vi "ClientForSingleDeviceDServer_05.vi"() -> ()   [LabVIEW 2014, in "examples.lvlib"]
uses:
  vis/tango_vi.llb/_DServerDevicePropertyToDouble.vi
  vis/tango_vi.llb/_DServerDevicePropertyToFloat.vi
  vis/tango_vi.llb/_DServerDevicePropertyToULong.vi
  vis/tango_vi.llb/_DServerDevicePropertyToLong.vi
  vis/tango_vi.llb/_DServerDevicePropertyToUShort.vi
  vis/tango_vi.llb/_DServerDevicePropertyToShort.vi
  vis/tango_vi.llb/_DServerDevicePropertyToBoolean.vi
  vis/tango_vi.llb/_DServerDevicePropertyToDoubleArray.vi
  vis/tango_vi.llb/_DServerDevicePropertyToFloatArray.vi
  vis/tango_vi.llb/_DServerDevicePropertyToShortArray.vi
  vis/tango_vi.llb/_DServerDevicePropertyToLongArray.vi
  vis/tango_vi.llb/_DServerDevicePropertyToString.vi
  vis/tango_vi.llb/_DServerDevicePropertyToStringArray.vi
  examples.lvlib
  vis/tango_vi.llb/tango.lvlib
panel:
  out "PropertyDevStringArray":string[](array[string])
  out "PropertyDevString":string
  out "PropertyDevLongArray":i32[](array[numeric])
  out "PropertyDevShortArray":i16[](array[numeric])
  out "PropertyDevFloatArray":dbl[](array[numeric])
  out "PropertyDevDoubleArray":dbl[](array[numeric])
  out "PropertyDevBoolean":bool=TRUE
  out "PropertyDevShort":i16
  out "PropertyDevUShort":u16
  out "PropertyDevLong":i32
  out "PropertyDevULong":u32
  out "PropertyDevFloat":sgl
  out "PropertyDevDouble":dbl
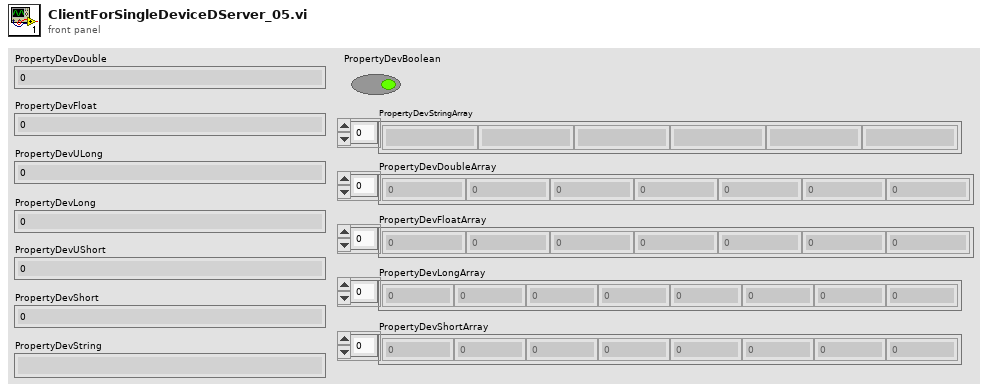
[diagram p1: front panel]
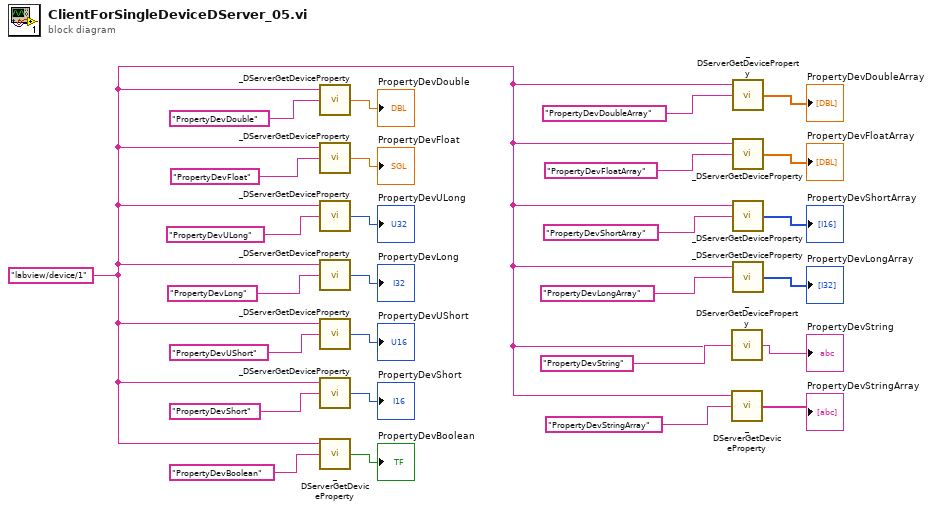
[diagram p0: block diagram]
diagram:
  w2 = "labview/device/1" ("device name")
  n1 = call-poly "_DServerGetDeviceProperty.vi"("property name"="PropertyDevDouble", "device name"=w2) -> ("property value"=→"PropertyDevDouble":dbl)  [unwired: 2 in, 1 out]
  n2 = call-poly "_DServerGetDeviceProperty.vi"("property name"="PropertyDevFloat", "device name"=w2) -> ("property value"=→"PropertyDevFloat":sgl)  [unwired: 2 in, 1 out]
  n3 = call-poly "_DServerGetDeviceProperty.vi"("property name"="PropertyDevULong", "device name"=w2) -> ("property value"=→"PropertyDevULong":u32)  [unwired: 2 in, 1 out]
  n4 = call-poly "_DServerGetDeviceProperty.vi"("property name"="PropertyDevLong", "device name"=w2) -> ("property value"=→"PropertyDevLong":i32)  [unwired: 2 in, 1 out]
  n5 = call-poly "_DServerGetDeviceProperty.vi"("property name"="PropertyDevUShort", "device name"=w2) -> ("property value"=→"PropertyDevUShort":u16)  [unwired: 2 in, 1 out]
  n6 = call-poly "_DServerGetDeviceProperty.vi"("property name"="PropertyDevShort", "device name"=w2) -> ("property value"=→"PropertyDevShort":i16)  [unwired: 2 in, 1 out]
  n7 = call-poly "_DServerGetDeviceProperty.vi"("property name"="PropertyDevBoolean", "device name"=w2) -> ("property value"=→"PropertyDevBoolean":bool)  [unwired: 2 in, 1 out]
  n8 = call-poly "_DServerGetDeviceProperty.vi"("property name"="PropertyDevString", "device name"=w2) -> ("propery value"=→"PropertyDevString":string)  [unwired: 2 in, 1 out]
  n9 = call-poly "_DServerGetDeviceProperty.vi"("property name"="PropertyDevStringArray", "device name"=w2) -> ("property value"=→"PropertyDevStringArray":string[])  [unwired: 2 in, 1 out]
  n10 = call-poly "_DServerGetDeviceProperty.vi"("property name"="PropertyDevDoubleArray", "device name"=w2) -> ("property value"=→"PropertyDevDoubleArray":dbl[])  [unwired: 2 in, 1 out]
  n11 = call-poly "_DServerGetDeviceProperty.vi"("property name"="PropertyDevFloatArray", "device name"=w2) -> ("property value"=→"PropertyDevFloatArray":sgl[])  [unwired: 2 in, 1 out]
  n12 = call-poly "_DServerGetDeviceProperty.vi"("property name"="PropertyDevShortArray", "device name"=w2) -> ("property value"=→"PropertyDevShortArray":i16[])  [unwired: 2 in, 1 out]
  n13 = call-poly "_DServerGetDeviceProperty.vi"("property name"="PropertyDevLongArray", "device name"=w2) -> ("property value"=→"PropertyDevLongArray":i32[])  [unwired: 2 in, 1 out]
